vi "Panther Dashboard--global.vi"() -> ()   [LabVIEW 2020, in "Panther Dashboard.lvlib"]
uses:
  Panther Dashboard.lvlib
panel:
  in  "DQMH_WAIT":string="DQMH_WAIT"
  in  "Module Timeout--constant.vi":string="Module Timeout--constant.vi"
  in  "DQMH_CUSTOM_TIMEOUT":string="DQMH_CUSTOM_TIMEOUT"
  in  "Target":string
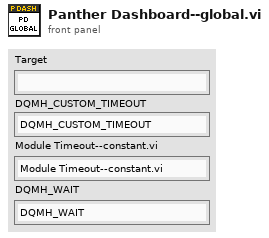
[diagram p1: front panel]
diagram:
